vi "Get Osc Support Samples.vi"(8 "error in (no error)":errorcluster, 10 "maxnum":i32, 11 "sample":u32[](array[numeric])=[0, 0, 0, 0, 0, 0, 0, 0, 0, 0, 0, 0, 0, 0, 0, 0, 0, 0, 0, 0, 0, 0, 0, 0, 0]) -> (0 "error out":errorcluster, 2 "function return":i32, 3 "sample out":u32[](array[numeric]))   [LabVIEW 2023, in "vmmsolib.lvlib"]
doc: "DLL_API int WINAPI GetOscSupportSamples(unsigned int* sample, int maxnum);"
uses:
  vmmsolib.lvlib
  vmmso.dll
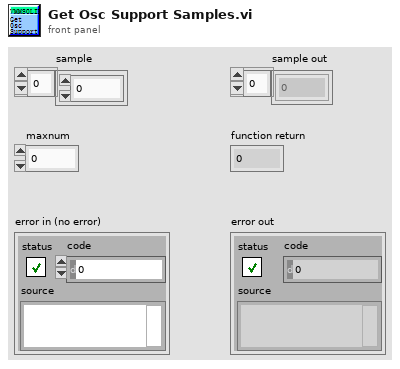
[diagram p1: front panel]
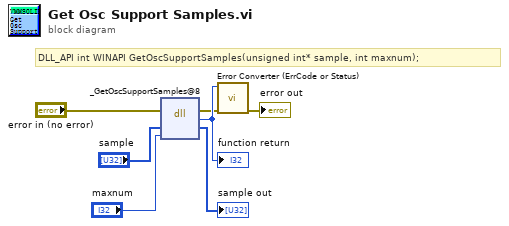
[diagram p0: block diagram]
diagram:
  # "DLL_API int WINAPI GetOscSupportSamples(unsigned int* sample, int maxnum);"
  n1 = dll-call lib="D:/VmMsoSDK/demo-Labview/2023/vmmsolib/vmmso.*" fn="_GetOscSupportSamples@8"(error in="error in (no error)", "sample"="sample", "maxnum"="maxnum") -> (error out=w2:errorcluster, w7:i32, "sample"=→"sample out":u32[])  [unwired: 3 in, 1 out]
  "function return" <- w7
  n2 = call "Error Converter (ErrCode or Status).vi"("error in (no error)"=w2, "error code"=w7) -> ("error out"=→"error out":errorcluster)  [unwired: 9 in]
